vi "Heizungsregelung.vi"() -> ()   [LabVIEW 2024]
uses:
  Treiber/Treiber Heizung/Thermostat Treiber.lvlib
  <vilib>/addons/control/pid/NI_PID_autopid.lvlib
panel:
  out "Thermometer":dbl(slide) scale=0.0..100.0
  out "Ventilstellung":dbl(slide) scale=0.0..100.0 scale format="%#_2f"
  out "Temperatur über der Zeit":cluster{timestamp[], dbl[]}(graph)
  in  "PID-Regler-Parameter":T1
  out "Fehlerausgang":errorcluster
  in  "Fehlereingang":errorcluster
  in  "Stop":bool
  in  "Thermostat":u32(knob) scale=0.0..3.0
  # "Standard 1\nIdealster Wert bisher 5"
  # "Standard 0,01\nIdealster Wert bisher 0,01"
  # "Standard 0\nIdealster Wert bisher 3"
  # "Bisher kleinste Hysterese: 0,41°C"
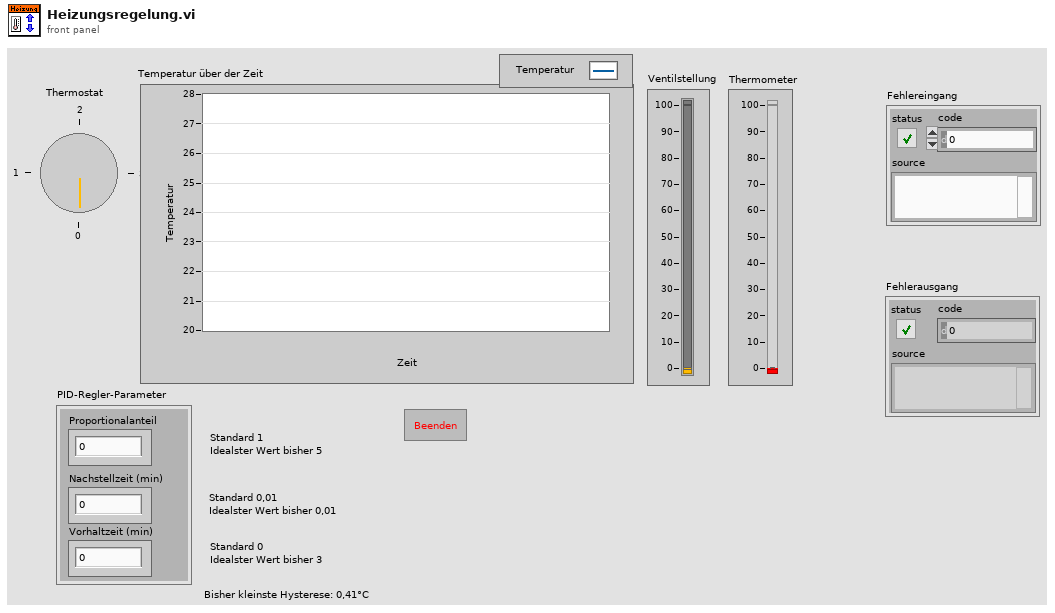
[diagram p1: front panel]
types:
  T1 = cluster{"Proportionalanteil":dbl, "Nachstellzeit (min)":dbl, "Vorhaltzeit (min)":dbl}
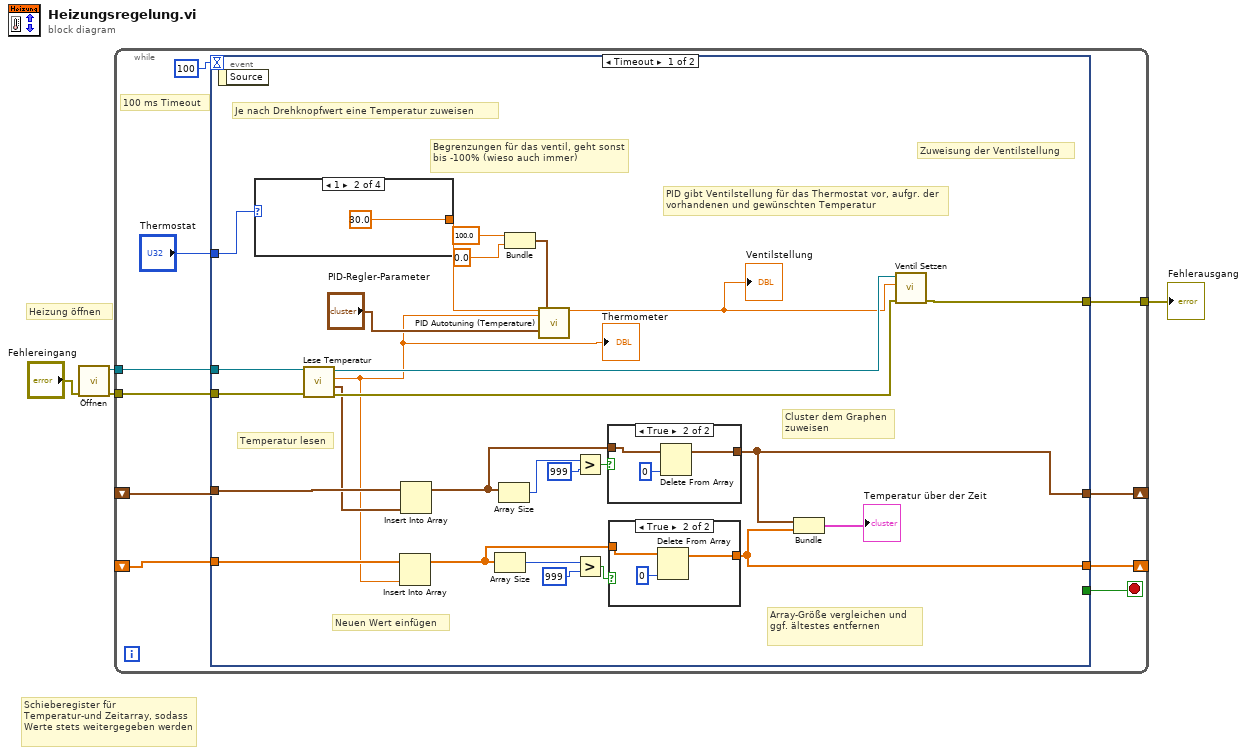
[diagram p0: block diagram]
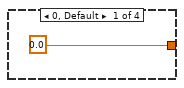
[diagram p4: hidden frame]
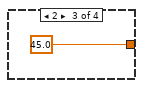
[diagram p5: hidden frame]
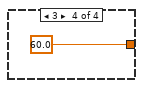
[diagram p6: hidden frame]
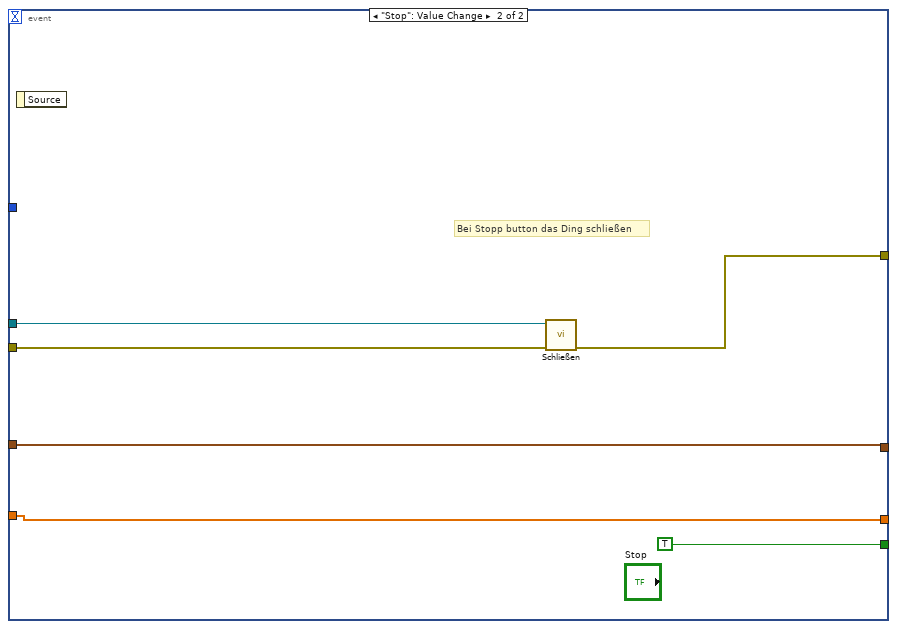
[diagram p7: hidden frame]
diagram:
  # "Schieberegister für Temperatur-und Zeitarray, sodass Werte stets weitergegeben werden"
  # "Heizung öffnen"
  n1 = call "Öffnen.vi"("Error In"="Fehlereingang") -> ("Error Out"=w2:errorcluster, "Verbindungs-ID"=w4:refnum<k16>)  [unwired: 9 in]
  n2 = while {
    tunnel: w4 -> [w12]
    tunnel: w2 -> [w11]
    tunnel: [w10] -> w1
    shift-right: [w7] -> _
    shift-left: _ -> [w8]
    shift-right: [w6] -> _
    shift-left: _ -> [w5]
    stop <- w13 stop-if-true
    # "100 ms Timeout"
    n3 = event shown="[0] Timeout" {
      selector: _ -> [_ _]
      dyn-events: _ -> [_ _]
      timeout: 100 -> [_ _]
      tunnel: [_ TRUE] -> w13
      tunnel: w12 -> [w40 w58]
      tunnel: w11 -> [w39 w57]
      tunnel: [w36 w56] -> w10
      tunnel: "Thermostat" -> [w41 _]
      tunnel: w8 -> [w30 w55]
      tunnel: [w20 w55] -> w7
      tunnel: [w21 w54] -> w6
      tunnel: w5 -> [w23 w54]
      event Timeout {
        # "Cluster dem Graphen zuweisen"
        # "Array-Größe vergleichen und ggf. ältestes entfernen"
        # "Neuen Wert einfügen"
        # "Zuweisung der Ventilstellung"
        # "PID gibt Ventilstellung für das Thermostat vor, aufgr. der vorhandenen und gewünschten Temperatur"
        # "Begrenzungen für das ventil, geht sonst bis -100% (wieso auch immer)"
        # "Temperatur lesen"
        # "Je nach Drehknopfwert eine Temperatur zuweisen"
        n4 = event-data() -> ()  [unwired: 1 in, 1 out]
        n5 = case shown="1" w41 {
          tunnel: [0.0 30.0 45.0 60.0] -> w35
          frame 0, Default {
          }
          frame 1 {
          }
          frame 2 {
          }
          frame 3 {
          }
        }
        n6 = call "Lese Temperatur.vi"("Error In"=w39, "Verbindungs-ID in"=w40) -> ("Error Out"=w37:errorcluster, "Zeitstempel-Bedienelement"=w18:timestamp, "Temperatur"=w15:dbl, "Verbindungs-ID out"=w38:refnum<k16>)  [unwired: 5 in, 1 out]
        "Thermometer" <- w15
        n7 = Insert Into Array(array=w23, new element=w15) -> (w22:dbl[])  [unwired: 1 in]
        n8 = Insert Into Array(array=w30, new element=w18) -> (w24:timestamp[])  [unwired: 1 in]
        n9 = Array Size(array=w22) -> (size(s)=w17:i32)
        n10 = Array Size(array=w24) -> (size(s)=w27:i32)
        n11 = Bundle(100.0, 0.0) -> (w32:cluster{dbl, dbl})  [unwired: 1 in]
        n12 = call <vilib>:"PID Autotuning (Temperature).vi"("desired temperature"=w35, "measured temperature"=w15, "PID gains in"="PID-Regler-Parameter", "output range"=w32) -> ("output"=w16:dbl)  [unwired: 12 in, 3 out]
        "Ventilstellung" <- w16
        n13 = Greater?(x=w27, y=999) -> (0:w29:bool)
        n14 = Greater?(x=w17, y=999) -> (0:w28:bool)
        n15 = case shown="True" w29 {
          tunnel: w24 -> [w46 w49]
          tunnel: [w46 w47] -> w20
          frame False {
          }
          frame True {
            n16 = Delete From Array(array=w49, index=0) -> (array with subset deleted=w47:timestamp[])  [unwired: 1 in, 1 out]
          }
        }
        n17 = case shown="True" w28 {
          tunnel: w22 -> [w42 w44]
          tunnel: [w42 w43] -> w21
          frame False {
          }
          frame True {
            n18 = Delete From Array(array=w44, index=0) -> (array with subset deleted=w43:dbl[])  [unwired: 1 in, 1 out]
          }
        }
        n19 = Bundle(w20, w21) -> (→"Temperatur über der Zeit":cluster{timestamp[], dbl[]})  [unwired: 1 in]
        n20 = call "Ventil Setzen.vi"("Error In"=w37, "Thermostat in %"=w16, "Verbindungs-ID in"=w38) -> ("Error Out"=w36:errorcluster)  [unwired: 7 in, 1 out]
      }
      event "Stop": Value Change {
        # "Bei Stopp button das Ding schließen"
        n21 = event-data() -> ()  [unwired: 1 in, 1 out]
        n22 = call "Schließen.vi"("Error In"=w57, "Verbindungs-ID"=w58) -> ("Error Out"=w56:errorcluster)  [unwired: 9 in]
      }
    }
  }
  "Fehlerausgang" <- w1
